vi "BOplus4ESP300 - Set DIO port A, B, C direction.vi"(3 "error in":errorcluster, 4 "Action":bool, 5 "Address / Port":i16=1 min=1 max=31 step=1) -> (0 "error out":errorcluster, 2 "Report the DIO port\ndirection configuration":string)   [LabVIEW 2014]
panel:
  in  "Port A":bool
  in  "Port B":bool
  # "Read"
  # "Write"
  # "Set digital I/O port A\nand B direction"
  # "Output"
  # "Output"
  # "Input"
  # "Input"
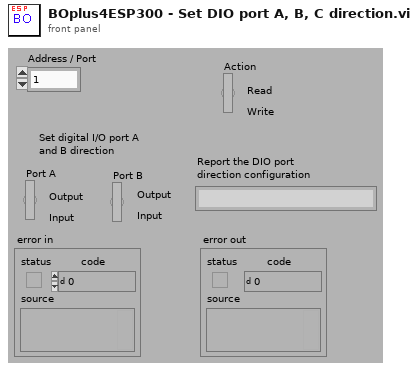
[diagram p1: front panel]
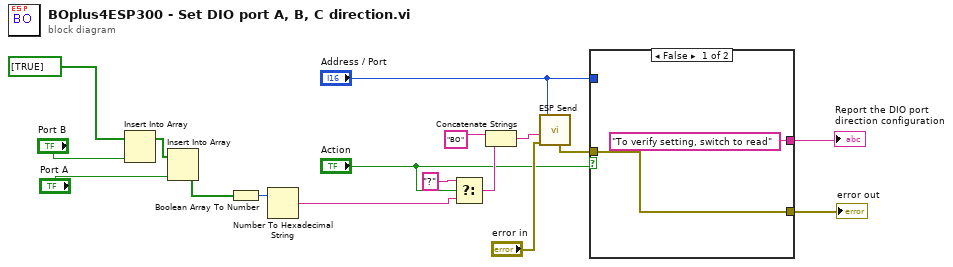
[diagram p0: block diagram]
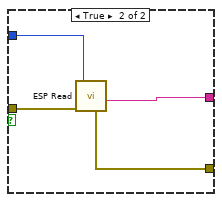
[diagram p2: hidden frame]
diagram:
  n1 = Insert Into Array(array=bool[] [TRUE] ("Input Array"), new element="Port B") -> (w5:bool[])  [unwired: 1 in]
  n2 = Insert Into Array(array=w5, new element="Port A") -> (w1:bool[])  [unwired: 1 in]
  n3 = Boolean Array To Number(Boolean array=w1) -> (number=w7:u32)
  n4 = Number To Hexadecimal String(2:w7) -> (0:w2:string)  [unwired: 1 in]
  n5 = Select(t="?", s="Action", f=w2) -> (s? t:f=w15:string)
  n6 = Concatenate Strings("BO" ("Substring"), w15) -> (w16:string)
  n7 = call "ESP Send.vi"("Address / Port"="Address / Port", "Command String"=w16, "error in"="error in") -> ("error out"=w10:errorcluster)  [unwired: 5 in]
  n8 = case shown="False" "Action" {
    tunnel: "Address / Port" -> [_ w23]
    tunnel: w10 -> [w19 w22]
    tunnel: [w19 w21] -> w9
    tunnel: ["To verify setting, switch to read" w20] -> w8
    frame False {
    }
    frame True {
      n9 = call "ESP Read.vi"("Address / Port"=w23, "error in"=w22) -> ("error out"=w21:errorcluster, "Response String"=w20:string)  [unwired: 5 in]
    }
  }
  "error out" <- w9
  "Report the DIO port\ndirection configuration" <- w8
